vi "Write Step Name.vi"(8 "error in (no error)":errorcluster, 10 "Step Name":string, 11 "Step Configuration in":refnum<class "Step Configuration.lvclass">) -> (0 "error out":errorcluster, 3 "Step Configuration out":refnum<class "Step Configuration.lvclass">)   [LabVIEW 2026, in "Measurement Actor.lvlib" / "Step Configuration.lvclass"]
uses:
  Step Configuration.lvclass
  Step Configuration.lvclass/Step Configuration.ctl
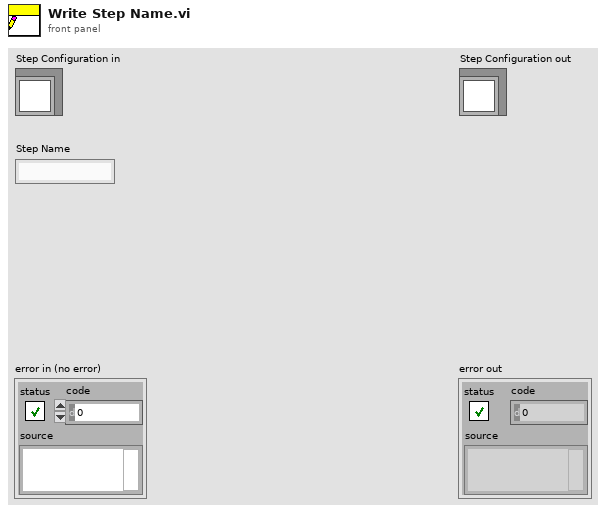
[diagram p1: front panel]
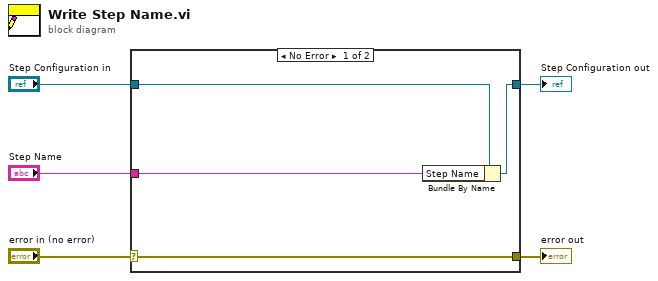
[diagram p0: block diagram]
diagram:
  n1 = case shown="No Error" "error in (no error)" {
    selector: "error in (no error)" -> [w9 w10]
    tunnel: [w9 w10] -> w4
    tunnel: [w7 w11] -> w2
    tunnel: "Step Configuration in" -> [w8 w11]
    tunnel: "Step Name" -> [w6 _]
    frame No Error {
      n2 = Bundle By Name(cluster=w8, "Step Name"=w6) -> (w7:refnum<class "Step Configuration.lvclass">)
    }
    frame Error {
    }
  }
  "error out" <- w4
  "Step Configuration out" <- w2
